vi "Periodic Tasks.vi"(8 "error in":errorcluster) -> ()   [LabVIEW 2012]
doc: "This VI runs in parallel to other tasks. It can contain as many user-defined periodic loops as you need. These can carry out PID or other sorts of timed response."
uses:
  <vilib>/Rock Robotics/SystemInterfaces/Utilities/FPGA_UtilitiesLED Source.ctl
  <vilib>/Rock Robotics/SystemInterfaces/Utilities/FPGA_UtilitiesLED State.ctl
  <vilib>/Rock Robotics/WPI/Relay/WPI_RelayValue.ctl
  <vilib>/Rock Robotics/WPI/Solenoid/WPI_SolenoidValue.ctl
  <vilib>/Rock Robotics/WPI/DriverStation/DriverStationLCD/WPI_DriverStationLCDLCDLine.ctl
  <vilib>/Rock Robotics/WPI/SafetyOutput/WPI_SafetyOutputConfigMenu.ctl
  Begin/Global Refnums.vi
  Begin/Global Variables.vi
  <vilib>/Rock Robotics/WPI/Solenoid/WPI_SolenoidSetEnum.vi
  <vilib>/Rock Robotics/WPI/Compressor/WPI_CompressorGetSetRefNum.vi
  Begin/Robot Global Data.vi
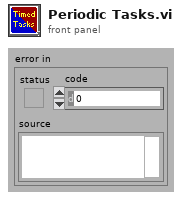
[diagram p1: front panel]
types:
  T1 = typedef "FPGA_UtilitiesLED State.ctl" = enum16{"Off", "On", "Toggle"}
  T2 = typedef "FPGA_UtilitiesLED Source.ctl" = enum16{"User LED", "FPGA LED"}
  T3 = typedef "WPI_SafetyOutputConfigMenu.ctl" = enum16{"Enable", "Disable"}
  T4 = typedef "WPI_SolenoidValue.ctl" = enum16{"Off", "On", "Forward", "Reverse"}
  T5 = typedef "WPI_DriverStationLCDLCDLine.ctl" = enum16{"Main - Line 1", "User - Line 2", "User - Line 3", "User - Line 4", "User - Line 5", "User - Line 6"}
  T6 = typedef "WPI_SolenoidDevRef.ctl" = cluster{"DevStatus":errorcluster, "Solenoid Module":T7, "Forward Solenoid Channel":T8, "Reverse Solenoid Channel":T8}
  T7 = typedef "FPGA_TypedefSolenoidModule.ctl" = enum16{"Solenoid Module 1", "Solenoid Module 2"}
  T8 = typedef "WPI_SolenoidChannel.ctl" = enum8{"Solenoid 1", "Solenoid 2", "Solenoid 3", "Solenoid 4", "Solenoid 5", "Solenoid 6", "Solenoid 7", "Solenoid 8", "Invalid"}
  T9 = typedef "WPI_MotorControlDeviceRef.ctl" = cluster{"DeviceStatus":errorcluster, "Type":enum16{"PWM", "CAN"}, "PWM":cluster{"Digital Module":T10, "PWM Channel":T11, "DeadBand":T12}, "CAN":cluster{"Device Number":u8, "Control Mode":T13, "Semaphore":T14, "Max Vout":dbl}, "Invert":bool, "TransformRef":T15, "InvTransformRef":T15}
  T10 = typedef "FPGA_TypedefDigitalModule.ctl" = enum16{"Digital Module 1", "Digital Module 2"}
  T11 = typedef "FPGA_DIOPWMChannel.ctl" = enum8{"PWM 1", "PWM 2", "PWM 3", "PWM 4", "PWM 5", "PWM 6", "PWM 7", "PWM 8", "PWM 9", "PWM 10", "Invalid"}
  T12 = typedef "WPI_PWMDeadband.ctl" = cluster{"Name":string, "maxPositivePwm":i32, "minPositivePwm":i32, "centerPwm":i32, "maxNegativePwm":i32, "minNegativePwm":i32, "angularRange":u16}
  T13 = typedef "WPI_CANJaguar_ControlMode.ctl" = enum8{"Percent VBus", "Current", "Speed", "Position", "Voltage"}
  T14 = typedef "Semaphore RefNum" = refnum<k1>
  T15 = typedef "WPI_PWMTransform_ConPane.ctl" = refnum<vi>
  T16 = typedef "WPI_RelayValue.ctl" = enum16{"Off", "On", "Forward", "Reverse"}
  T17 = typedef "WPI_CompressorDevRef.ctl" = cluster{"DevStatus":errorcluster, "DigitalInputDevRef":T18, "RelayDevRef":T20}
  T18 = typedef "WPI_DigitalInputDevRef.ctl" = cluster{"DevStatus":errorcluster, "DIO Channel":T19, "Digital Module":T10}
  T19 = typedef "FPGA_DIOChannel.ctl" = enum8{"DIO 1", "DIO 2", "DIO 3", "DIO 4", "DIO 5", "DIO 6", "DIO 7", "DIO 8", "DIO 9", "DIO 10", "DIO 11", "DIO 12", "DIO 13", "DIO 14", "Invalid"}
  T20 = typedef "WPI_RelayDevRef.ctl" = cluster{"DevStatus":errorcluster, "Relay Channel":T21, "Digital Module":T10, "Relay Direction":T22}
  T21 = typedef "FPGA_DIORelayChannel.ctl" = enum8{"Relay 1", "Relay 2", "Relay 3", "Relay 4", "Relay 5", "Relay 6", "Relay 7", "Relay 8", "Invalid"}
  T22 = typedef "WPI_RelayDirection.ctl" = enum16{"Both directions", "Forward only", "Reverse only"}
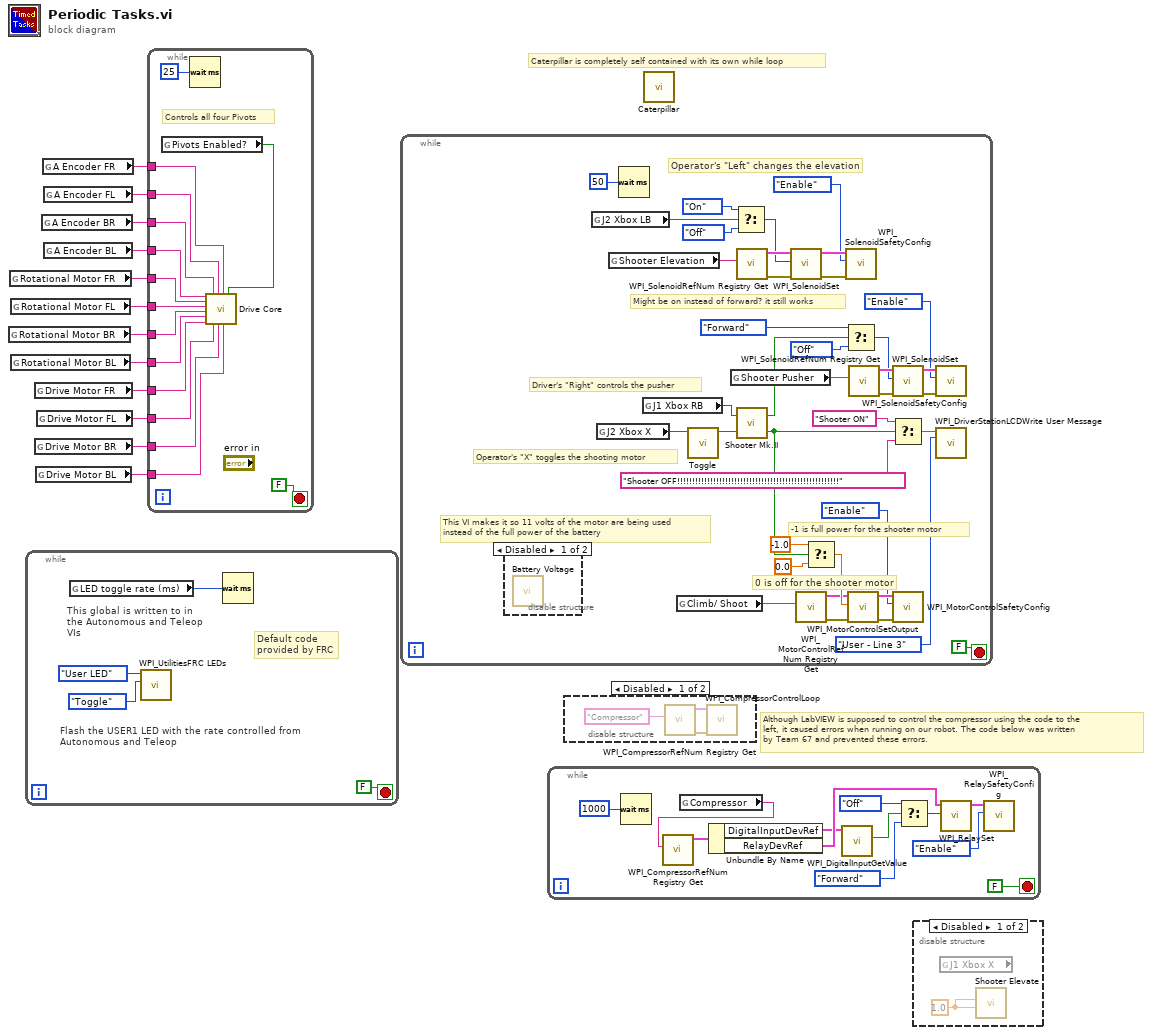
[diagram p0: block diagram]
diagram:
  # "Although LabVIEW is supposed to control the compressor using the code to the\nleft, it caused errors when running on our robot. The code below was written\nby Team 67 and prevented these errors."
  # "Caterpillar is completely self contained with its own while loop"
  n1 = global read "Global Refnums.vi" "Rotational Motor BR"() -> (w3:string)
  n2 = global read "Global Refnums.vi" "Rotational Motor FR"() -> (w4:string)
  n3 = global read "Global Refnums.vi" "Rotational Motor FL"() -> (w1:string)
  n4 = global read "Global Refnums.vi" "Rotational Motor BL"() -> (w2:string)
  n5 = while {
    stop <- FALSE stop-if-true
    # "Default code\nprovided by FRC"
    # "This global is written to in the Autonomous and Teleop VIs"
    # "Flash the USER1 LED with the rate controlled from Autonomous and Teleop"
    n6 = global read "Robot Global Data.vi" "LED toggle rate (ms)"() -> (w13:u32)
    n7 = call <vilib>:"WPI_UtilitiesFRC LEDs.vi"("State"=FPGA_UtilitiesLED_State."Toggle", "LED Type"=FPGA_UtilitiesLED_Source."User LED") -> ()  [unwired: 1 in, 9 out]
    n8 = Wait (ms)(milliseconds to wait=w13) -> ()  [unwired: 1 out]
  }
  n9 = global read "Global Refnums.vi" "Drive Motor FR"() -> (w8:string)
  n10 = global read "Global Refnums.vi" "Drive Motor BR"() -> (w7:string)
  n11 = global read "Global Refnums.vi" "Drive Motor BL"() -> (w6:string)
  n12 = global read "Global Refnums.vi" "Drive Motor FL"() -> (w5:string)
  n13 = global read "Global Refnums.vi" "A Encoder BR"() -> (w11:string)
  n14 = global read "Global Refnums.vi" "A Encoder FR"() -> (w12:string)
  n15 = global read "Global Refnums.vi" "A Encoder FL"() -> (w9:string)
  n16 = global read "Global Refnums.vi" "A Encoder BL"() -> (w10:string)
  n17 = while {
    tunnel: w12 -> [w30]
    tunnel: w11 -> [w28]
    tunnel: w10 -> [w27]
    tunnel: w9 -> [w29]
    tunnel: w8 -> [w22]
    tunnel: w7 -> [w20]
    tunnel: w6 -> [w19]
    tunnel: w5 -> [w21]
    tunnel: w4 -> [w26]
    tunnel: w3 -> [w24]
    tunnel: w2 -> [w23]
    tunnel: w1 -> [w25]
    stop <- FALSE stop-if-true
    # "Controls all four Pivots"
    n18 = global read "Global Variables.vi" "Pivots Enabled?"() -> (w17:bool)
    n19 = Wait (ms)(milliseconds to wait=u32 25) -> ()  [unwired: 1 out]
    n20 = call "Drive Core.vi"("A Encoder BL"=w27, "Rotational Motor FR"=w26, "Rotational Motor FL"=w25, "Rotational Motor BR"=w24, "Rotational Motor BL"=w23, "Drive Motor FR"=w22, "A Encoder BR"=w28, "Drive Motor FL"=w21, "A Encoder FL"=w29, "Drive Motor BR"=w20, "A Encoder FR"=w30, "Drive Motor BL"=w19, "Enabled?"=w17) -> ()  [unwired: 7 in]
  }
  n21 = while {
    stop <- FALSE stop-if-true
    # "This VI makes it so 11 volts of the motor are being used\ninstead of the full power of the battery"
    # "0 is off for the shooter motor"
    # "-1 is full power for the shooter motor"
    # "Operator's \"X\" toggles the shooting motor"
    # "Driver's \"Right\" controls the pusher"
    # "Might be on instead of forward? it still works"
    # "Operator's \"Left\" changes the elevation"
    n22 = disable-structure shown="Disabled" {
      frame Disabled {
        n23 = call "Battery Voltage.vi"() -> ()  [unwired: 1 out]
      }
      frame Enabled {
      }
    }
    n24 = global read "Global Variables.vi" "J2 Xbox LB"() -> (w50:bool)
    n25 = global read "Global Variables.vi" "J2 Xbox X"() -> (w54:bool)
    n26 = global read "Global Refnums.vi" "Shooter Elevation"() -> (w58:string)
    n27 = Wait (ms)(milliseconds to wait=u32 50) -> ()  [unwired: 1 out]
    n28 = global read "Global Variables.vi" "J1 Xbox RB"() -> (w40:bool)
    n29 = global read "Global Refnums.vi" "Climb/ Shoot"() -> (w34:string)
    n30 = call "Toggle.vi"("Boolean"=w54) -> ("Toggled"=w41:bool)  [unwired: 10 in]
    n31 = global read "Global Refnums.vi" "Shooter Pusher"() -> (w57:string)
    n32 = Select(t=WPI_SolenoidValue."On" ("Value"), s=w50, f=WPI_SolenoidValue."Off" ("Value")) -> (s? t:f=w53:T4)
    n33 = call <vilib>:"WPI_SolenoidRefNum Registry Get.vi"("refnum name"=w58) -> ("error out"=w62:errorcluster, "SolenoidDevRef"=w63:T6)  [unwired: 9 in]
    n34 = call "Shooter Mk.II.vi"("Motor"=w41, "Fire"=w40) -> ("Shooter On"=w33:bool, "Extend Shooter"=w43:bool)
    n35 = call-poly <vilib>:"WPI_SolenoidSet.vi"("error in (no error)"=w62, "Value"=w53, "SolenoidDevRef"=w63) -> ("error out"=w60:errorcluster, "SolenoidDevRef"=w61:T6)  [unwired: 7 in]
    n36 = call <vilib>:"WPI_MotorControlRefNum Registry Get.vi"("refnum name"=w34) -> ("error out"=w38:errorcluster, "MotorControlDevRef"=w39:T9)  [unwired: 9 in]
    n37 = Select(t=-1.0, s=w33, f=0.0) -> (s? t:f=w56:dbl)
    n38 = call <vilib>:"WPI_SolenoidSafetyConfig.vi"("error in (no error)"=w60, "mode"=WPI_SafetyOutputConfigMenu."Enable", "SolenoidDevRef"=w61) -> ()  [unwired: 7 in, 2 out]
    n39 = Select(t=WPI_SolenoidValue."Forward", s=w43, f=WPI_SolenoidValue."Off" ("Value")) -> (s? t:f=w48:T4)
    n40 = call <vilib>:"WPI_MotorControlSetOutput.vi"("error in (no error)"=w38, "Output"=w56, "MotorControlDevRef"=w39) -> ("error out"=w36:errorcluster, "MotorControlDevRef"=w37:T9)  [unwired: 6 in, 1 out]
    n41 = call <vilib>:"WPI_SolenoidRefNum Registry Get.vi"("refnum name"=w57) -> ("error out"=w69:errorcluster, "SolenoidDevRef"=w70:T6)  [unwired: 9 in]
    n42 = call-poly <vilib>:"WPI_SolenoidSet.vi"("error in (no error)"=w69, "Value"=w48, "SolenoidDevRef"=w70) -> ("error out"=w68:errorcluster, "SolenoidDevRef"=w67:T6)  [unwired: 7 in]
    n43 = Select(t="Shooter ON", s=w33, f="Shooter OFF!!!!!!!!!!!!!!!!!!!!!!!!!!!!!!!!!!!!!!!!!!!!!!!!!!!!!!") -> (s? t:f=w45:string)
    n44 = call <vilib>:"WPI_MotorControlSafetyConfig.vi"("error in (no error)"=w36, "mode"=WPI_SafetyOutputConfigMenu."Enable", "MotorControlDevRef"=w37) -> ()  [unwired: 7 in, 2 out]
    n45 = call <vilib>:"WPI_SolenoidSafetyConfig.vi"("error in (no error)"=w68, "mode"=WPI_SafetyOutputConfigMenu."Enable", "SolenoidDevRef"=w67) -> ()  [unwired: 7 in, 2 out]
    n46 = call <vilib>:"WPI_DriverStationLCDWrite User Message.vi"("line text"=w45, "line"=WPI_DriverStationLCDLCDLine."User - Line 3") -> ()  [unwired: 13 in, 1 out]
  }
  n47 = while {
    stop <- FALSE stop-if-true
    n48 = Wait (ms)(milliseconds to wait=u32 1000) -> ()  [unwired: 1 out]
    n49 = global read "Global Refnums.vi" "Compressor"() -> (w71:string)
    n50 = call <vilib>:"WPI_CompressorRefNum Registry Get.vi"("refnum name"=w71) -> ("CompressorDevRef"=w82:T17)  [unwired: 9 in, 1 out]
    n51 = Unbundle By Name(w82) -> ("DigitalInputDevRef"=w80:T18, "RelayDevRef"=w81:T20)
    n52 = call <vilib>:"WPI_DigitalInputGetValue.vi"("DigitalInputDevRef"=w80) -> ("Value"=w79:bool)  [unwired: 8 in, 2 out]
    n53 = Select(t=WPI_RelayValue."Off" ("RelayValue"), s=w79, f=WPI_RelayValue."Forward" ("RelayValue")) -> (s? t:f=w74:T16)
    n54 = call <vilib>:"WPI_RelaySet.vi"("RelayValue"=w74, "RelayDevRef"=w81) -> ("RelayDevRef"=w76:T20)  [unwired: 8 in, 1 out]
    n55 = call <vilib>:"WPI_RelaySafetyConfig.vi"("mode"=WPI_SafetyOutputConfigMenu."Enable", "RelayDevRef"=w76) -> ()  [unwired: 8 in, 2 out]
  }
  n56 = disable-structure shown="Disabled" {
    frame Disabled {
      n57 = call <vilib>:"WPI_CompressorRefNum Registry Get.vi"("refnum name"="Compressor") -> ("error out"=w85:errorcluster, "CompressorDevRef"=w84:T17)  [unwired: 9 in]
      n58 = call <vilib>:"WPI_CompressorControlLoop.vi"("error in (no error)"=w85, "CompressorDevRef"=w84) -> ()  [unwired: 10 in]
    }
    frame Enabled {
    }
  }
  n59 = call "Caterpillar.vi"() -> ()  [unwired: 12 in]
  n60 = disable-structure shown="Disabled" {
    frame Disabled {
      w86 = 1.0 ("Lowering time (s)")
      n61 = global read "Global Variables.vi" "J1 Xbox X"() -> ()  [unwired: 1 out]
      n62 = call "Shooter Elevate.vi"("Elevation time (s)"=w86, "Lowering time (s)"=w86) -> ()  [unwired: 8 in, 2 out]
    }
    frame Enabled {
    }
  }
